vi "MultiChanAtoD.vi"(6 "Array Input":dbl[](array[numeric]), 8 "Chans":u32, 9 "Samples":dbl) -> (0 "u8Array":u8[][](array[numeric]), 1 "u16Array":u16[][](array[numeric]), 2 "u32Array":u32[][](array[numeric]), 3 "sCnSu32":u32[](array[numeric]), 4 "sCnSu16":u16[](array[numeric]), 5 "sCnSu8":u8[](array[numeric]))   [LabVIEW 2010]
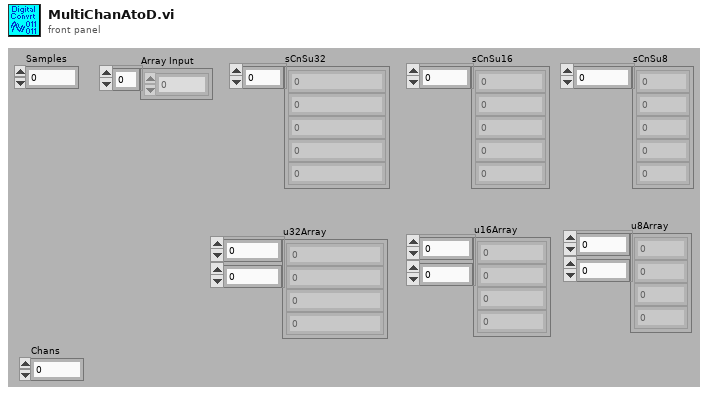
[diagram p1: front panel]
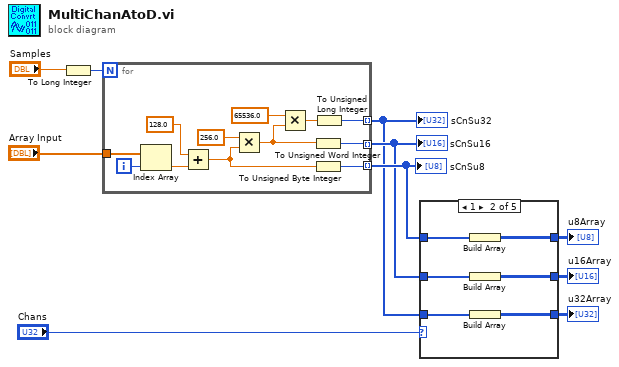
[diagram p0: block diagram]
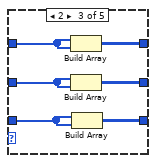
[diagram p3: hidden frame]
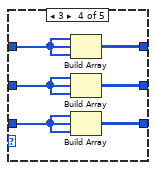
[diagram p4: hidden frame]
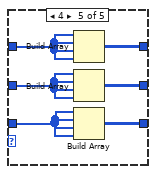
[diagram p5: hidden frame]
diagram:
  n1 = To Long Integer(number="Samples") -> (32bit integer=w10:i32)
  n2 = for {
    N: w10 -> [_]
    tunnel: "Array Input" -> [w21]
    tunnel: [w18] -> w7 mode=indexing
    tunnel: [w20] -> w6 mode=indexing
    tunnel: [w14] -> w5 mode=indexing
    i -> [w22]
    n3 = Index Array(array=w21, index=w22) -> (element=w13:dbl)
    n4 = Add(x=128.0, y=w13) -> (x+y=w12:dbl)
    n5 = Multiply(x=256.0, y=w12) -> (x*y=w16:dbl)
    n6 = Multiply(x=65536.0, y=w16) -> (x*y=w17:dbl)
    n7 = To Unsigned Word Integer(number=w16) -> (unsigned 16bit integer=w20:u16)
    n8 = To Unsigned Byte Integer(number=w12) -> (unsigned 8bit integer=w18:u8)
    n9 = To Unsigned Long Integer(number=w17) -> (unsigned 32bit integer=w14:u32)
  }
  "sCnSu16" <- w6
  "sCnSu8" <- w7
  "sCnSu32" <- w5
  n10 = case shown="1" "Chans" {
    tunnel: w7 -> [_ w28 w34 w40 w44]
    tunnel: [_ w27 w32 w37 w45] -> w3
    tunnel: w6 -> [_ w26 w33 w39 w43]
    tunnel: [_ w25 w31 w38 w46] -> w2
    tunnel: w5 -> [_ w24 w29 w35 w42]
    tunnel: [_ w23 w30 w36 w41] -> w1
    frame 0, Default {
    }
    frame 1 {
      n11 = Build Array(w28) -> (w27:u8[][])
      n12 = Build Array(w26) -> (w25:u16[][])
      n13 = Build Array(w24) -> (w23:u32[][])
    }
    frame 2 {
      n14 = Build Array(w34, w34) -> (w32:u8[][])
      n15 = Build Array(w33, w33) -> (w31:u16[][])
      n16 = Build Array(w29, w29) -> (w30:u32[][])
    }
    frame 3 {
      n17 = Build Array(w40, w40, w40) -> (w37:u8[][])
      n18 = Build Array(w39, w39, w39) -> (w38:u16[][])
      n19 = Build Array(w35, w35, w35) -> (w36:u32[][])
    }
    frame 4 {
      n20 = Build Array(w44, w44, w44, w44) -> (w45:u8[][])
      n21 = Build Array(w43, w43, w43, w43) -> (w46:u16[][])
      n22 = Build Array(w42, w42, w42, w42) -> (w41:u32[][])
    }
  }
  "u8Array" <- w3
  "u16Array" <- w2
  "u32Array" <- w1
